vi "GL_MeasData_to.vi"(4 "Temp":bool, 6 "RD+":i32 caption="Count", 10 "Ack":string, 11 "HEAD":T1={"File"=[refnum], "Idx"=[], "dT"=0.5, "Hd"=4096, "Rd"=14, "Start"=[timestamp(3519879471 s since 1904-01-01)], "Trig"=[timestamp(3519879472 s since 1904-01-01)], "Stop"=[timestamp(3519940623 s since 1904-01-01)], "FirstPos"=[], "Count"=[120609], "Color"=[27836, 4765252, 11010216, 14712848], "Label"=["CH1", "CH2", "CH3", "CH4"], "INP"=["CH1", "CH2", "CH3", "CH4"], "H"=[5.0, 5.0, 5.0, 5.0], "L"=[-5.0, -5.0, -5.0, -5.0], "Fmt"=["%.;%+0.3f V", "%.;%+0.3f V", "%.;%+0.3f V", "%.;%+0.3f V"], "Unit"=["", "", "", ""], "SEL"=[0, 1, 2, 3], "Byte"=[-2, -2, -2, -2], "Pos"=[], "Bit"=[], "Flg"=[], "Gain"=[], "Offset"=[0.01, 0.01, 0.01, 0.01], "CH"=[0, 0, 0, 0], "Opt"={"Mode"=0, "TUNIT"=enum."CELS"}, "TYPE"=enum."GBD", "Comp"=[], "Temp"=[]} {"FirstPos" format="%<%x %.3X>T"; "Stop" format="%<%x %.3X>T"; "Trig" format="%<%x %.3X>T"; "Start" format="%<%x %.3X>T"}) -> (0 "Fmt":string[](array[string]), 1 "Status":u8[][](array[numeric]), 2 "Alarm":u8[][](array[numeric]), 3 "Data":dbl[][](array[numeric]), 5 "dT":dbl, 7 "Count":i32)   [LabVIEW 2017]
uses:
  Amp_Param.ctl
  Driver/TempConv.dll
panel:
  # "ALL"
  # "GBD"
  # "CSV"
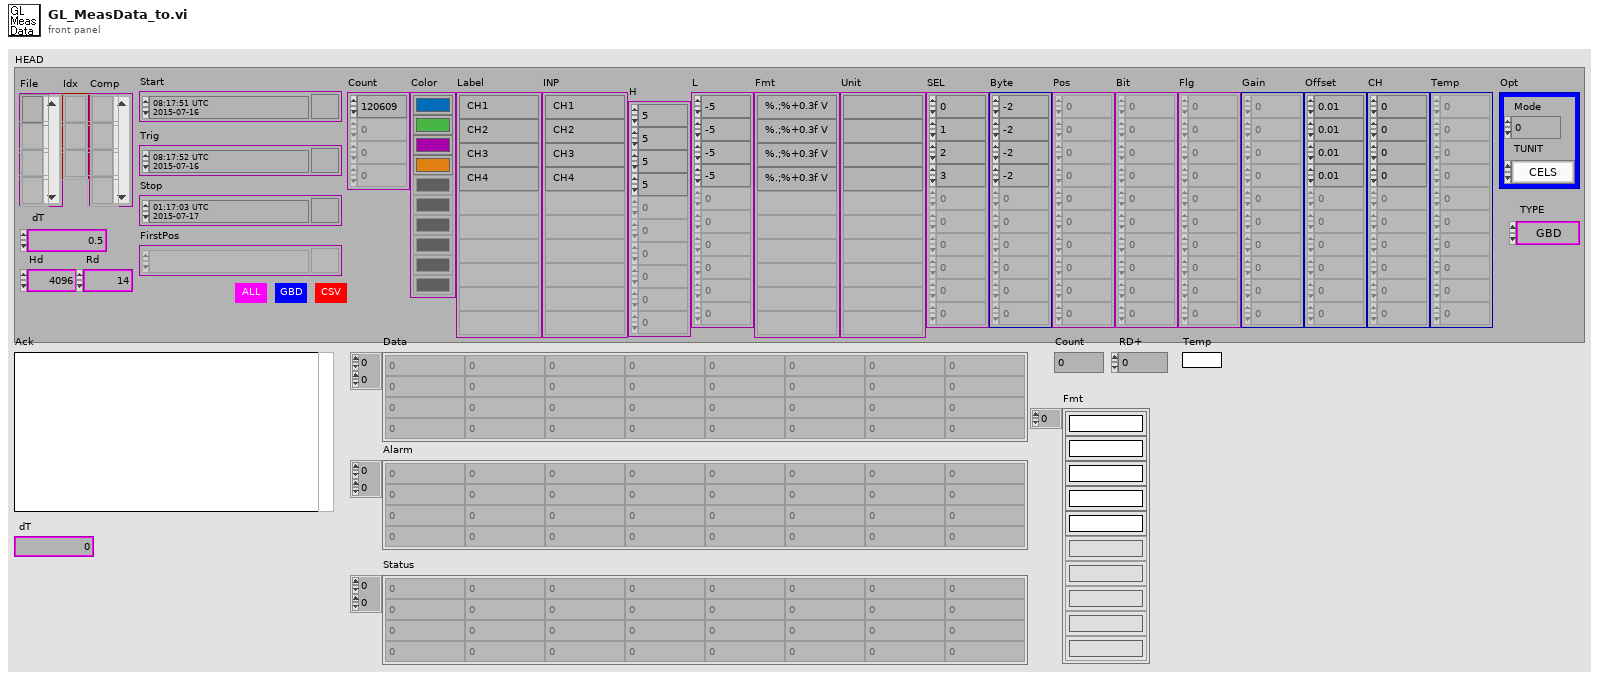
[diagram p1: front panel]
types:
  T1 = typedef "Amp_Param.ctl" = cluster{"File":refnum<file>[], "Idx":refnum<file>[], "dT":dbl, "Hd":i32, "Rd":i32, "Start":timestamp[], "Trig":timestamp[], "Stop":timestamp[], "FirstPos":timestamp[], "Count":i64[], "Color":u32[], "Label":string[], "INP":string[], "H":dbl[], "L":dbl[], "Fmt":string[], "Unit":string[], "SEL":i32[], "Byte":i32[], "Pos":i32[], "Bit":i32[], "Flg":i32[], "Gain":dbl[], "Offset":dbl[], "CH":i32[], "Opt":cluster{"Mode":i32, "TUNIT":enum16{"CELS", "FAHR"}}, "TYPE":enum16{"GBD", "CSV"}, "Comp":refnum<file>[], "Temp":i32[]}
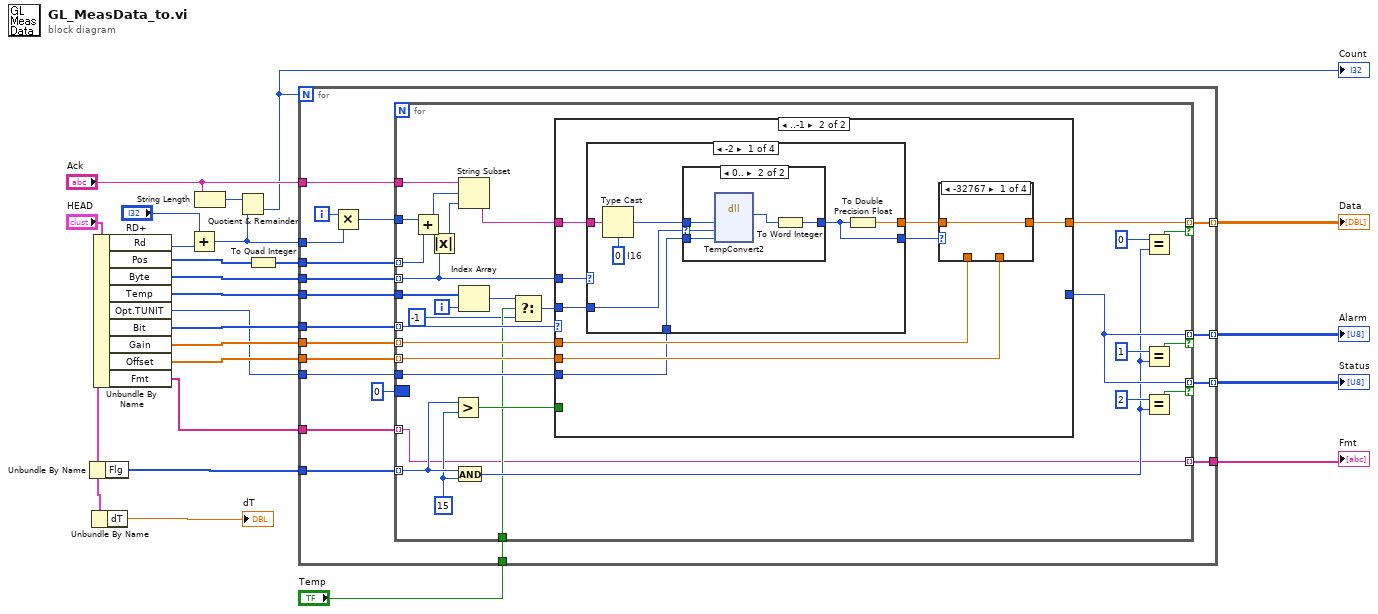
[diagram p0: block diagram]
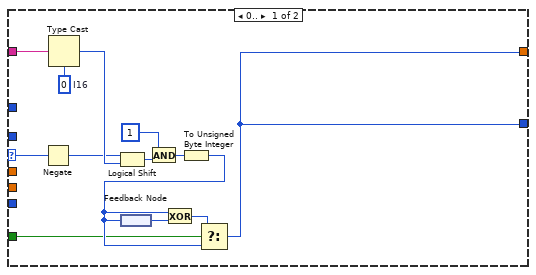
[diagram p2: hidden frame]
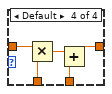
[diagram p5: hidden frame]
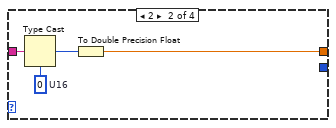
[diagram p7: hidden frame]
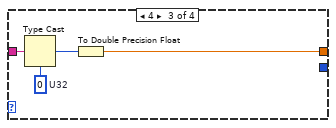
[diagram p8: hidden frame]
diagram:
  n1 = Unbundle By Name("HEAD") -> ("Flg"=w11:i32[])
  n2 = Unbundle By Name("HEAD") -> ("dT"=→"dT":dbl)
  n3 = Unbundle By Name("HEAD") -> ("Rd"=w18:i32, "Pos"=w23:i32[], "Byte"=w22:i32[], "Temp"=w8:i32[], "Opt.TUNIT"=w7:enum16{"CELS", "FAHR"}, "Bit"=w21:i32[], "Gain"=w14:dbl[], "Offset"=w13:dbl[], "Fmt"=w2:string[])
  n4 = Add(x="RD+", y=w18) -> (x+y=w6:i32)
  n5 = String Length(string="Ack") -> (length=w19:i32)
  n6 = Quotient & Remainder(x=w19, y=w6) -> (floor(x/y)=w9:i32)  [unwired: 1 out]
  "Count" <- w9
  n7 = To Quad Integer(1:w23) -> (0:w3:i64[])
  n8 = for {
    N: w9 -> [_]
    tunnel: "Ack" -> [w32]
    tunnel: w6 -> [w30]
    tunnel: w3 -> [w41]
    tunnel: w22 -> [w40]
    tunnel: w21 -> [w39]
    tunnel: [w38] -> w17 mode=indexing
    tunnel: w14 -> [w37]
    tunnel: w13 -> [w36]
    tunnel: [w35] -> w16 mode=indexing
    tunnel: w11 -> [w34]
    tunnel: [w33] -> w10 mode=indexing
    tunnel: w8 -> [w28]
    tunnel: w7 -> [w27]
    tunnel: "Temp" -> [w26]
    tunnel: [w24] -> w1
    tunnel: w2 -> [w25]
    i -> [w42]
    n9 = Multiply(x=w42, y=w30) -> (x*y=w31:i32)
    n10 = for {
      tunnel: w32 -> [w70]
      tunnel: w31 -> [w72]
      tunnel: w41 -> [w71] mode=indexing
      tunnel: w40 -> [w68] mode=indexing
      tunnel: w39 -> [w63] mode=indexing
      tunnel: [w64] -> w38 mode=indexing if=w60
      tunnel: w37 -> [w66] mode=indexing
      tunnel: w36 -> [w65] mode=indexing
      tunnel: [w56] -> w35 mode=indexing if=w62
      tunnel: w34 -> [w53] mode=indexing
      tunnel: [w56] -> w33 mode=indexing if=w61
      border: u8 0 -> [_]
      tunnel: w28 -> [w50]
      tunnel: w27 -> [w49]
      tunnel: w26 -> [w45]
      tunnel: w25 -> [w43] mode=indexing
      tunnel: [w43] -> w24 mode=indexing
      i -> [w47]
      w52 = 15 ("x")
      n11 = Add(x=w72, y=w71) -> (x+y=w69:i64)
      n12 = Absolute Value(x=w68) -> (abs(x)=w67:i32)
      n13 = Greater?(x=w53, y=w52) -> (0:w51:bool)
      n14 = And(x=w53, y=w52) -> (x .and. y?=w54:i32)
      n15 = String Subset(string=w70, offset (0)=w69, length (rest)=w67) -> (substring=w55:string)
      n16 = Index Array(array=w50, index=w47) -> (element=w48:i32)
      n17 = Select(t=w48, s=w45, f=-1) -> (s? t:f=w46:i32)
      n18 = case shown="..-1" w63 {
        selector: w63 -> [w78 _]
        tunnel: w68 -> [_ w94]
        tunnel: w55 -> [w84 w93]
        tunnel: w66 -> [_ w90]
        tunnel: w65 -> [_ w89]
        tunnel: [w73 w88] -> w64
        tunnel: [w73 _] -> w56
        tunnel: w51 -> [w75 _]
        tunnel: w46 -> [_ w87]
        tunnel: w49 -> [_ w86]
        frame 0.. {
          w85 = i16 0  # I16
          n19 = Negate(x=w78) -> (-x=w82:i32)
          n20 = Type Cast(type=w85, x=w84) -> (*(type *) &x=w83:i16)
          n21 = Logical Shift(y=w82, x=w83) -> (x << y=w80:i16)
          n22 = feedback #1() -> (w77:u8)
          n23 = And(x=i16 1 ("y"), y=w80) -> (x .and. y?=w81:i16)
          n24 = To Unsigned Byte Integer(number=w81) -> (unsigned 8bit integer=w76:u8)
          n25 = feedback-in #1(w76) -> ()
          n26 = Exclusive Or(1:w77, 2:w76) -> (0:w74:u8)
          n27 = Select(t=w74, s=w75, f=w76) -> (s? t:f=w73:u8)
        }
        frame ..-1 {
          n28 = case shown="-2" w94 {
            tunnel: w93 -> [w108 w117 w121 _]
            tunnel: [w107 w116 w120 _] -> w92
            tunnel: [w105 _ _ _] -> w91
            tunnel: w87 -> [w104 _ _ _]
            tunnel: w86 -> [w103 _ _ _]
            frame -2 {
              w109 = i16 0  # I16
              n29 = Type Cast(type=w109, x=w108) -> (*(type *) &x=w106:i16)
              n30 = case shown="0.." w104 {
                selector: w104 -> [_ w115]
                tunnel: w106 -> [w110 w112]
                tunnel: w103 -> [_ w114]
                tunnel: [w110 w111] -> w105
                frame ..-1 {
                }
                frame 0.. {
                  n31 = dll-call lib="D:/src/LabVIEW/GL860/JP/LabView VI/Driver/TempConv.dll" fn="TempConvert2"("AdData"=w112, "TcCode"=w115, "TempUnit"=w114) -> ("return type"=w113:i32)  [unwired: 6 in, 2 out]
                  n32 = To Word Integer(number=w113) -> (16bit integer=w111:i16)
                }
              }
              n33 = To Double Precision Float(number=w105) -> (double precision float=w107:dbl)
            }
            frame 2 {
              w118 = u16 0  # U16
              n34 = Type Cast(type=w118, x=w117) -> (*(type *) &x=w119:u16)
              n35 = To Double Precision Float(number=w119) -> (double precision float=w116:dbl)
            }
            frame 4 {
              w122 = u32 0  # U32
              n36 = Type Cast(type=w122, x=w121) -> (*(type *) &x=w123:u32)
              n37 = To Double Precision Float(number=w123) -> (double precision float=w120:dbl)
            }
            frame Default {
            }
          }
          n38 = case shown="-32767" w91 {
            tunnel: w92 -> [w95 w96 w97 w101]
            tunnel: [w95 w96 w97 w100] -> w88
            tunnel: w89 -> [_ _ _ w99]
            tunnel: w90 -> [_ _ _ w98]
            frame -32767 {
            }
            frame 32764 {
            }
            frame 32765 {
            }
            frame Default {
              n39 = Multiply(x=w101, y=w98) -> (x*y=w102:dbl)
              n40 = Add(x=w102, y=w99) -> (x+y=w100:dbl)
            }
          }
        }
      }
      n41 = Equal?(x=0, y=w54) -> (x = y?=w60:bool)
      n42 = Equal?(x=1, y=w54) -> (x = y?=w62:bool)
      n43 = Equal?(x=2, y=w54) -> (x = y?=w61:bool)
    }
  }
  "Data" <- w17
  "Alarm" <- w16
  "Status" <- w10
  "Fmt" <- w1
